vi "XP2i.vi"(4 "error in":T12, 7 "Command":T13) -> (0 "error out":T12, 3 "Response":T10)   [LabVIEW 2018]
uses:
  MOKO_LabViewLibrary/MokoLowLevel/MokoLowLovelControl/MLLC_Command.ctl
  MOKO_LabViewLibrary/MokoLowLevel/MokoLowLovelControl/MLLC_Error.ctl
  MOKO_LabViewLibrary/MokoLowLevel/MokoLowLovelControl/MLLC_Mode.ctl
  MOKO_LabViewLibrary/MokoLowLevel/MokoLowLovelControl/MLLC_Response.ctl
  MOKO_LabViewLibrary/MokoLowLevel/MokoLowLovelControl/MLLC_DriverName.ctl
  MOKO_LabViewLibrary/MokoLowLevel/MokoLowLovelControl/MLLC_ResponseInit.ctl
  MOKO_LabViewLibrary/MokoLowLevel/MokoLowLovelControl/MLLC_Request.ctl
  MOKO_LabViewLibrary/MokoLowLevel/MokoLowLovelControl/MLLC_ErrorCode.ctl
  MOKO_LabViewLibrary/MokoLowLevel/MokoLowLovelControl/MLLC_DriverConnectCluster.ctl
  MOKO_LabViewLibrary/MokoLowLevel/MokoLowLovelControl/MLLC_InterfaceType.ctl
  MOKO_LabViewLibrary/MokoLowLevel/MokoLowLovelControl/MLLC_OpenedSession.ctl
  MOKO_LabViewLibrary/MokoLowLevel/MokoLowLovelControl/MLLC_InterfaceSettings.ctl
  MOKO_LabViewLibrary/MokoLowLevel/MokoLowLovelControl/MLLC_InterfaceKind.ctl
  MOKO_LabViewLibrary/MokoLowLevel/MokoLowLovelControl/MLLC_Rs232Settings.ctl
panel:
  in  "DriverSettings":cluster{"DriverConnect":T1}={"DriverConnect"={"InterfaceType"=enum."VISA", "OpenedSession"="COM4", "InterfaceSettings"={"Interface"=enum."RS232", "EOS 4 read"=enum."Default (=EOS 4 write)", "EOS 4 write"=enum."CR (\\r)", "TMO, ms"=2000, "Sett"=variant(cluster{"Baud Rate":u32, "Data Bits":u16, "Parity":u16, "Stop Bits":u16, "Flow Control":u16, "Eho":bool} {"Baud Rate"=75, "Data Bits"=0, "Parity"=0, "Stop Bits"=0, "Flow Control"=0, "Eho"=FALSE})}}}
  in  "Error Code":T6=5420
  in  "Request":T7="?MOD"
  in  "ResponseInit":T8="XP2I"
  in  "Driver Name":T9="Crystal XP2"
  in  "Mode":T11=enum."Check"
  # "XP2i"
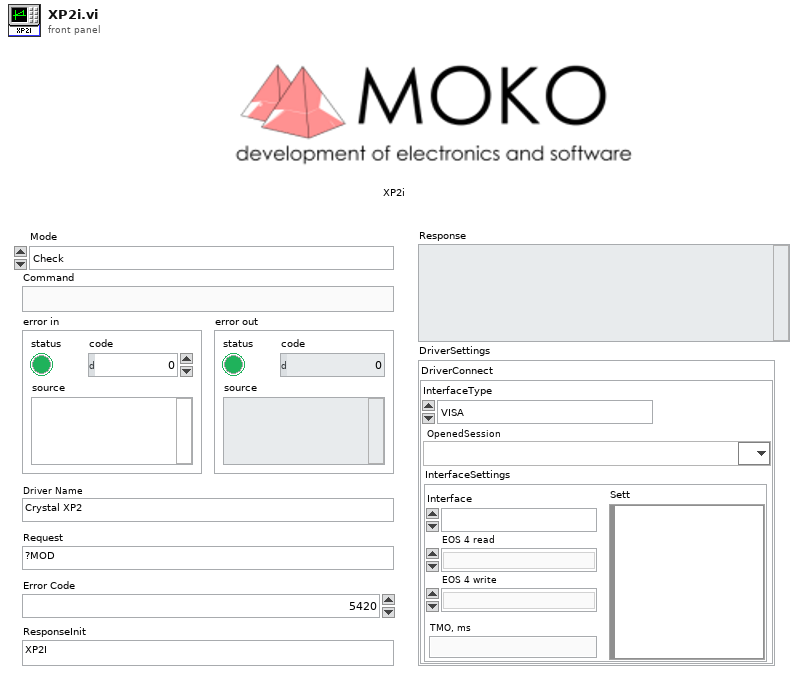
[diagram p1: front panel]
types:
  T1 = typedef "MLLC_DriverConnectCluster.ctl" = cluster{"InterfaceType":T2, "OpenedSession":T3, "InterfaceSettings":T4}
  T2 = typedef "MLLC_InterfaceType.ctl" = enum16{"VISA", "Prologix USB-GPIB"}
  T3 = typedef "MLLC_OpenedSession.ctl" = refnum<visa-resource-name>
  T4 = typedef "MLLC_InterfaceSettings.ctl" = cluster{"Interface":T5, "EOS 4 read":enum16{"Default (=EOS 4 write)", "CR (\\r)", "LF (\\n)", "None"}, "EOS 4 write":enum16{"CR+LF (\\r\\n)", "CR (\\r)", "LF (\\n)", "None"}, "TMO, ms":i32, "Sett":variant}
  T5 = typedef "MLLC_InterfaceKind.ctl" = enum16{"RS232", "GPIB", "USB", "Ethernet", "another"}
  T6 = typedef "MLLC_ErrorCode.ctl" = u32
  T7 = typedef "MLLC_Request.ctl" = string
  T8 = typedef "MLLC_ResponseInit.ctl" = string
  T9 = typedef "MLLC_DriverName.ctl" = string
  T10 = typedef "MLLC_Response.ctl" = string
  T11 = typedef "MLLC_Mode.ctl" = enum16{"get", "set", "close", "Init", "Check"}
  T12 = typedef "MLLC_Error.ctl" = errorcluster
  T13 = typedef "MLLC_Command.ctl" = string
  T14 = typedef "MLLC_Rs232Settings.ctl" = cluster{"Baud Rate":u32, "Data Bits":u16, "Parity":u16, "Stop Bits":u16, "Flow Control":u16, "Eho":bool}
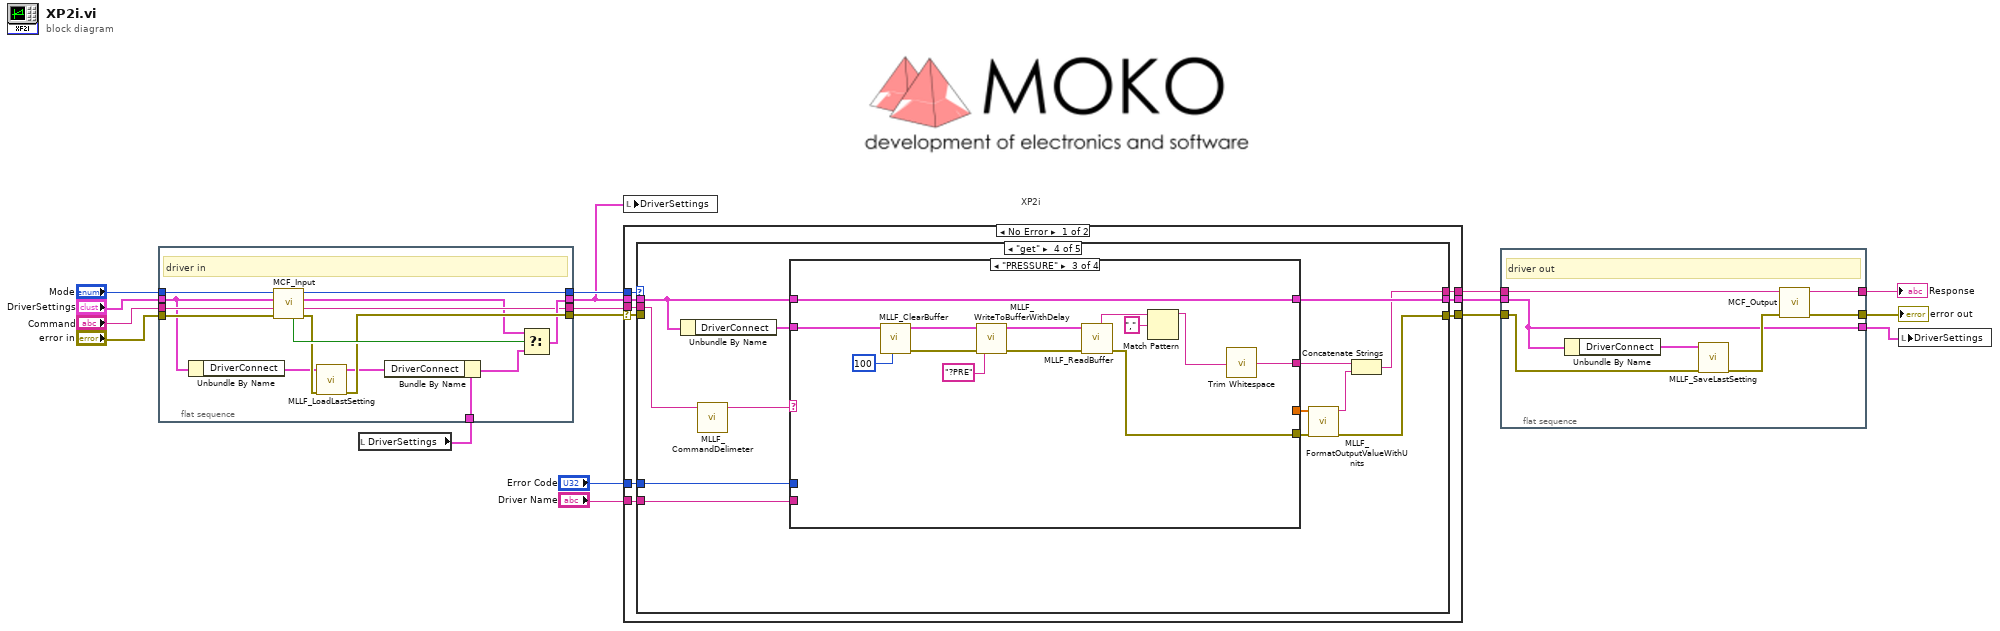
[diagram p0: block diagram]
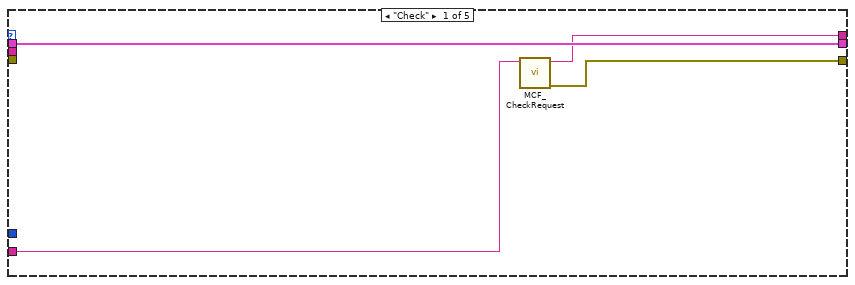
[diagram p2: hidden frame]
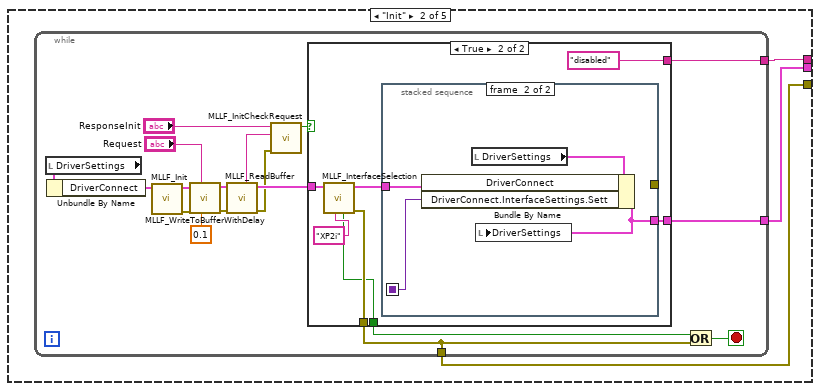
[diagram p3: hidden frame]
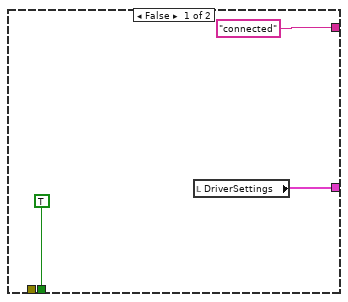
[diagram p4: hidden frame]
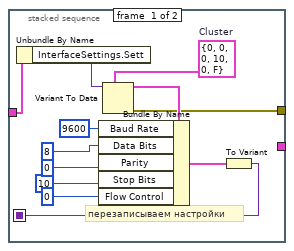
[diagram p5: hidden frame]
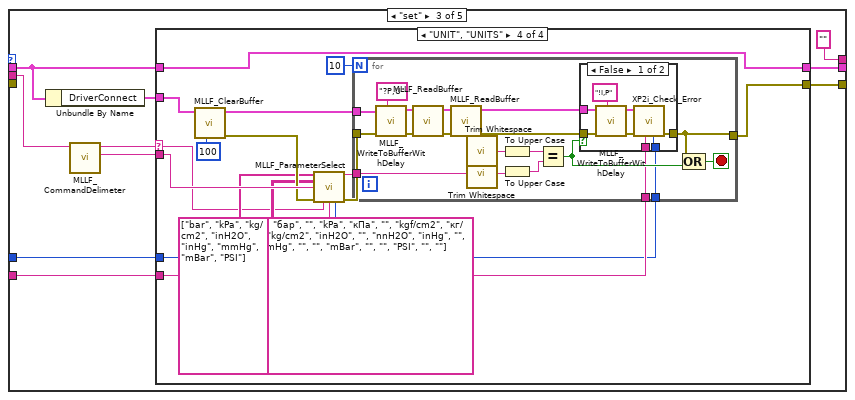
[diagram p6: hidden frame]
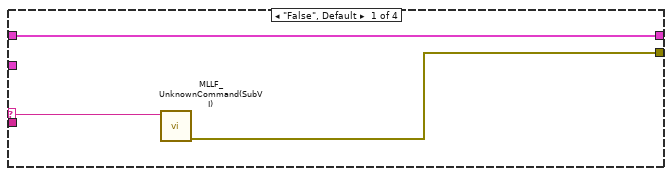
[diagram p7: hidden frame]
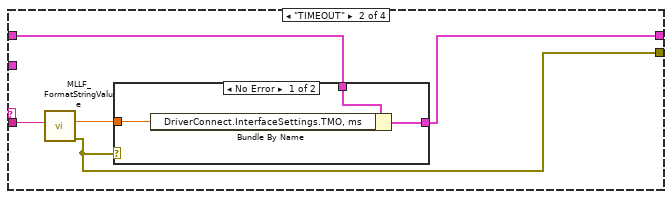
[diagram p8: hidden frame]
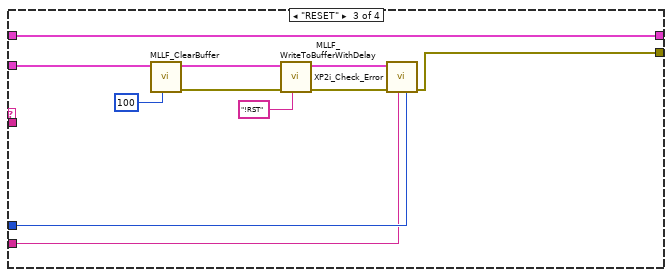
[diagram p10: hidden frame]
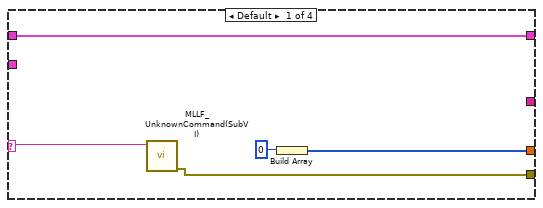
[diagram p12: hidden frame]
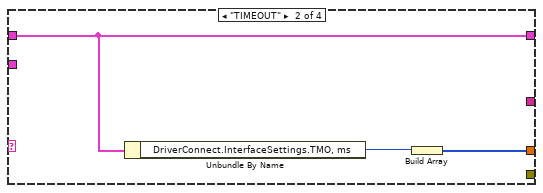
[diagram p13: hidden frame]
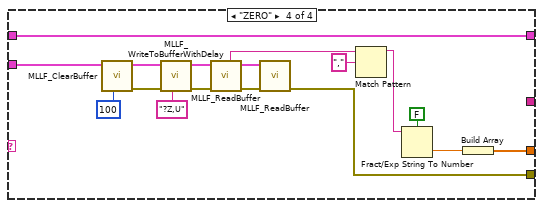
[diagram p14: hidden frame]
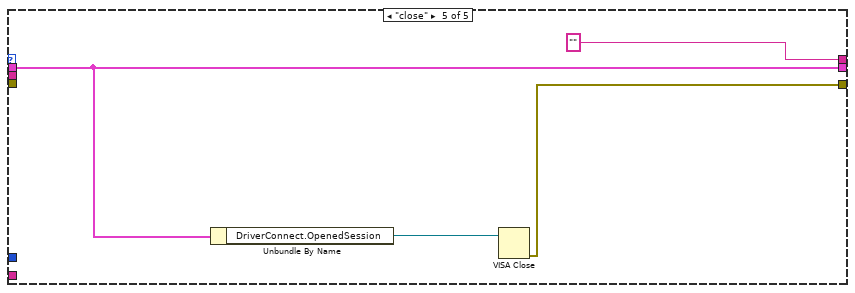
[diagram p15: hidden frame]
diagram:
  # "XP2i"
  n1 = flat-sequence {
    tunnel: [w26] -> w9
    tunnel: [w31] -> w11
    tunnel: "Command" -> [w28]
    tunnel: "Mode" -> [w30]
    tunnel: "DriverSettings" -> [w22]
    tunnel: w12 -> [w20]
    tunnel: "error in" -> [w25]
    tunnel: [w24] -> w10
    tunnel: [w23] -> w8
    frame #0 {
      # "driver in"
      n2 = Unbundle By Name(w22) -> ("DriverConnect"=w21:T1)
      n3 = call "MCF_Input.vi"("error in (no error)"=w25, "Command"=w28, "Mode"=w30) -> ("error out"=w27:errorcluster, "Command out"=w23:string, "Mode out"=w31:T11, "Boolean"=w29:bool)  [unwired: 5 in]
      n4 = call "MLLF_LoadLastSetting.vi"("Error In"=w27, "DriverConnectCluster in"=w21) -> ("Error Out"=w26:errorcluster, "DriverConnectCluster out"=w19:T1)  [unwired: 8 in]
      n5 = Bundle By Name(cluster=w20, "DriverConnect"=w19) -> (w18:cluster{"DriverConnect":T1})
      n6 = Select(t=w22, s=w29, f=w18) -> (s? t:f=w24:cluster{"DriverConnect":T1})
    }
  }
  n7 = local read "DriverSettings"() -> (w12:cluster{"DriverConnect":T1})
  n8 = local write "DriverSettings"(w10) -> ()
  n9 = case shown="No Error" w9 {
    selector: w9 -> [w37 w225]
    tunnel: [w32 w225] -> w1
    tunnel: w11 -> [w40 _]
    tunnel: [w39 _] -> w7
    tunnel: w8 -> [w38 _]
    tunnel: w10 -> [w34 w224]
    tunnel: "Error Code" -> [w36 _]
    tunnel: "Driver Name" -> [w35 _]
    tunnel: [w33 w224] -> w6
    frame No Error {
      n10 = case shown="\"get\"" w40 {
        tunnel: [w42 w47 "" ("Output String") w177 "" ("Output String")] -> w39
        tunnel: w38 -> [_ _ w94 w170 _]
        tunnel: w37 -> [_ _ _ _ _]
        tunnel: w36 -> [_ _ w101 w180 _]
        tunnel: w35 -> [w43 _ w98 w179 _]
        tunnel: w34 -> [w44 _ w100 w181 w222]
        tunnel: [w44 w46 w99 w178 w222] -> w33
        tunnel: [w41 w45 w97 w171 w221] -> w32
        frame "Check" {
          n11 = call "MCF_CheckRequest.vi"("Driver Name"=w43) -> ("Error Out"=w41:errorcluster, "Output String"=w42:string)  [unwired: 9 in]
        }
        frame "Init" {
          n12 = while {
            tunnel: [w60] -> w45
            tunnel: [w57] -> w47
            tunnel: [w56] -> w46
            stop <- w62 stop-if-true
            n13 = local read "DriverSettings"() -> (w50:cluster{"DriverConnect":T1})
            n14 = Unbundle By Name(w50) -> ("DriverConnect"=w49:T1)
            n15 = call "MLLF_Init.vi"("DriverConnect in"=w49) -> ("Error Out"=w64:errorcluster, "DriverConnect out"=w63:T1)  [unwired: 7 in]
            n16 = call "MLLF_WriteToBufferWithDelay.vi"("Delay Time ( 0,05 s)"=0.1 ("Delay Time (s)"), "Command"="Request", "Error In"=w64, "DriverConnect in"=w63) -> ("Error Out"=w59:errorcluster, "DriverConnect out"=w48:T1)  [unwired: 6 in]
            n17 = call "MLLF_ReadBuffer.vi"("Error In"=w59, "DriverConnect in"=w48) -> ("Error Out"=w54:errorcluster, "DriverConnect out"=w65:T1, "String"=w55:string)  [unwired: 6 in]
            n18 = call "MLLF_InitCheckRequest.vi"("error in (no error)"=w54, "Answer"=w55, "Response Init"="ResponseInit") -> ("Design"=w53:bool)  [unwired: 7 in, 1 out]
            n19 = case shown="True" w53 {
              tunnel: w65 -> [_ w74]
              tunnel: [TRUE w70] -> w61
              tunnel: [_ w75] -> w60
              tunnel: ["connected" "disabled"] -> w57
              tunnel: [w66 w69] -> w56
              frame False {
                n20 = local read "DriverSettings"() -> (w66:cluster{"DriverConnect":T1})
              }
              frame True {
                n21 = call "MLLF_InterfaceSelection.vi"("Driver Name"="XP2i" ("String"), "DriverConnect in"=w74) -> ("error out"=w75:T12, "DriverConnect out"=w73:T1, "stop init?"=w70:bool)  [unwired: 7 in]
                n22 = stacked-sequence {
                  seq-local: [w79 _] -> [_ w88]
                  tunnel: w73 -> [w77 w89]
                  tunnel: [w80 _] -> _
                  tunnel: [_ w90] -> w69
                  frame #0 {
                    w81 = T14 {"Baud Rate"=0, "Data Bits"=0, "Parity"=0, "Stop Bits"=10, "Flow Control"=0, "Eho"=FALSE}  # Cluster
                    # "перезаписываем настройки"
                    n23 = Unbundle By Name(w77) -> ("InterfaceSettings.Sett"=w76:variant)
                    n24 = Variant To Data(type=w81, Variant=w76) -> (data=w82:T14, error out=w80:errorcluster)  [unwired: 1 in]
                    n25 = Bundle By Name(cluster=w82, "Baud Rate"=u32 9600, "Data Bits"=u16 8 ("Serial Settings:Data Bits"), "Parity"=u16 0 ("Serial Settings:Parity"), "Stop Bits"=u16 10 ("Serial Settings:Stop Bits"), "Flow Control"=u16 0 ("Serial Settings:Flow Control")) -> (w87:T14)
                    n26 = To Variant(anything=w87) -> (Variant=w79:variant)
                  }
                  frame #1 {
                    n27 = local read "DriverSettings"() -> (w91:cluster{"DriverConnect":T1})
                    n28 = Bundle By Name(cluster=w91, "DriverConnect"=w89, "DriverConnect.InterfaceSettings.Sett"=w88) -> (w90:cluster{"DriverConnect":T1})
                    n29 = local write "DriverSettings"(w90) -> ()
                  }
                }
              }
            }
            n30 = Or(x=w61, y=w60) -> (x .or. y?=w62:bool)
          }
        }
        frame "set" {
          n31 = Unbundle By Name(w100) -> ("DriverConnect"=w95:T1)
          n32 = call "MLLF_CommandDelimeter.vi"("command with param"=w94) -> ("param 1"=w92:string, "command"=w93:string)  [unwired: 7 in, 2 out]
          n33 = case shown="\"UNIT\", \"UNITS\"" w93 {
            selector: w93 -> [w103 _ _ w125]
            tunnel: w92 -> [_ w107 _ w137]
            tunnel: w101 -> [_ _ w122 w135]
            tunnel: w100 -> [w104 w108 w124 w128]
            tunnel: [w104 w109 w124 w128] -> w99
            tunnel: w98 -> [_ _ w121 w136]
            tunnel: w95 -> [_ _ w115 w127]
            tunnel: [w102 w105 w114 w126] -> w97
            frame "False", Default {
              n34 = call "MLLF_UnknownCommand(SubVI).vi"("Unknown command"=w103) -> ("error out"=w102:errorcluster)  [unwired: 10 in]
            }
            frame "TIMEOUT" {
              n35 = call "MLLF_FormatStringValue.vi"("String Value"=w107) -> ("error out"=w105:T12, "number"=w106:dbl)  [unwired: 8 in, 1 out]
              n36 = case shown="No Error" w105 {
                tunnel: [w112 w113] -> w109
                tunnel: w108 -> [w111 w113]
                tunnel: w106 -> [w110 _]
                frame No Error {
                  n37 = Bundle By Name(cluster=w111, "DriverConnect.InterfaceSettings.TMO, ms"=w110) -> (w112:cluster{"DriverConnect":T1})
                }
                frame Error {
                }
              }
            }
            frame "RESET" {
              n38 = call "MLLF_ClearBuffer.vi"("Timeout"=u32 100, "DriverConnect in"=w115) -> ("Error Out"=w119:errorcluster, "DriverConnect out"=w118:T1)  [unwired: 6 in, 1 out]
              n39 = call "MLLF_WriteToBufferWithDelay.vi"("Command"="!RST" ("String"), "Error In"=w119, "DriverConnect in"=w118) -> ("Error Out"=w117:errorcluster, "DriverConnect out"=w123:T1)  [unwired: 7 in]
              n40 = call "XP2i_Check_Error.vi"("Error Code"=w122, "Driver Name"=w121, "Error In"=w117, "DriverConnect in"=w123) -> ("Error Out"=w114:errorcluster)  [unwired: 6 in, 1 out]
            }
            frame "UNIT", "UNITS" {
              n41 = call "MLLF_ClearBuffer.vi"("Timeout"=u32 100, "DriverConnect in"=w127) -> ("Error Out"=w134:errorcluster, "DriverConnect out"=w138:T1)  [unwired: 6 in, 1 out]
              n42 = call "MLLF_ParameterSelect.vi"("Command to equipment"=string[] ["bar", "kPa", "kg/cm2", "inH2O", "inHg", "mmHg", "mBar", "PSI"] ("Parameters 2 equipment"), "Names"=string[][] [["bar", "бар", ""], ["kPa", "кПа", ""], ["kgf/cm2", "кг/см2", "kg/cm2"], ["inH2O", "", "nnH2O"], ["inHg", "", ""], ["mmHg", "", ""], ["mBar", "", ""], ["PSI", "", ""]], "Input"=w137, "Error In"=w134, "Command"=w125, "Driver Name"=w136, "Error Code"=w135) -> ("Choice"=w132:string, "Error Out"=w133:errorcluster)  [unwired: 7 in]
              n43 = for {
                N: 10 -> [_]
                tunnel: w138 -> [w149]
                tunnel: [w143] -> w126
                tunnel: w132 -> [w147]
                tunnel: w136 -> [w141]
                tunnel: w135 -> [w140]
                tunnel: w133 -> [w148]
                stop <- w155 stop-if-true
                n44 = call "MLLF_WriteToBufferWithDelay.vi"("Command"="?P,U" ("String"), "Error In"=w148, "DriverConnect in"=w149) -> ("Error Out"=w151:errorcluster, "DriverConnect out"=w158:T1)  [unwired: 7 in]
                n45 = call "MLLF_ReadBuffer.vi"("Error In"=w151, "DriverConnect in"=w158) -> ("Error Out"=w154:errorcluster, "DriverConnect out"=w153:T1)  [unwired: 6 in, 1 out]
                n46 = call "MLLF_ReadBuffer.vi"("Error In"=w154, "DriverConnect in"=w153) -> ("Error Out"=w144:errorcluster, "DriverConnect out"=w145:T1, "String"=w152:string)  [unwired: 6 in]
                n47 = call <vilib>:"Trim Whitespace.vi"("string"=w152) -> ("trimmed string"=w150:string)  [unwired: 1 in]
                n48 = call <vilib>:"Trim Whitespace.vi"("string"=w147) -> ("trimmed string"=w146:string)  [unwired: 1 in]
                n49 = To Upper Case(1:w150) -> (0:w157:string)
                n50 = To Upper Case(1:w146) -> (0:w156:string)
                n51 = Equal?(x=w157, y=w156) -> (x = y?=w142:bool)
                n52 = case shown="False" w142 {
                  tunnel: w145 -> [w164 _]
                  tunnel: w144 -> [w163 w168]
                  tunnel: [w162 w168] -> w143
                  tunnel: w141 -> [w161 _]
                  tunnel: w140 -> [w160 _]
                  frame False {
                    n53 = call "MLLF_WriteToBufferWithDelay.vi"("Command"="!I,P" ("String"), "Error In"=w163, "DriverConnect in"=w164) -> ("Error Out"=w165:errorcluster, "DriverConnect out"=w166:T1)  [unwired: 7 in]
                    n54 = call "XP2i_Check_Error.vi"("Error Code"=w160, "Driver Name"=w161, "Error In"=w165, "DriverConnect in"=w166) -> ("Error Out"=w162:errorcluster)  [unwired: 6 in, 1 out]
                  }
                  frame True {
                  }
                }
                n55 = Compound Arithmetic op=OR(w143, w142) -> (w155:bool)
              }
            }
          }
        }
        frame "get" {
          n56 = Unbundle By Name(w181) -> ("DriverConnect"=w172:T1)
          n57 = call "MLLF_CommandDelimeter.vi"("command with param"=w170) -> ("command"=w169:string)  [unwired: 7 in, 3 out]
          n58 = case shown="\"PRESSURE\"" w169 {
            selector: w169 -> [w183 _ _ _]
            tunnel: [w182 _ w198 w212] -> w176
            tunnel: w180 -> [_ _ _ _]
            tunnel: [w186 w189 w202 w219] -> w178
            tunnel: w181 -> [w186 w189 w202 w219]
            tunnel: [w184 w187 _ w216] -> w175
            tunnel: w179 -> [_ _ _ _]
            tunnel: [_ _ w193 _] -> w173
            tunnel: w172 -> [_ _ w190 w203]
            frame Default {
              n59 = call "MLLF_UnknownCommand(SubVI).vi"("Unknown command"=w183) -> ("error out"=w182:errorcluster)  [unwired: 10 in]
              n60 = Build Array(0 ("TimeOut")) -> (w184:i32[])
            }
            frame "TIMEOUT" {
              n61 = Unbundle By Name(w189) -> ("DriverConnect.InterfaceSettings.TMO, ms"=w188:i32)
              n62 = Build Array(w188) -> (w187:i32[])
            }
            frame "PRESSURE" {
              n63 = call "MLLF_ClearBuffer.vi"("Timeout"=u32 100, "DriverConnect in"=w190) -> ("Error Out"=w199:errorcluster, "DriverConnect out"=w200:T1)  [unwired: 6 in, 1 out]
              n64 = call "MLLF_WriteToBufferWithDelay.vi"("Command"="?PRE" ("String"), "Error In"=w199, "DriverConnect in"=w200) -> ("Error Out"=w192:errorcluster, "DriverConnect out"=w197:T1)  [unwired: 7 in]
              n65 = call "MLLF_ReadBuffer.vi"("Error In"=w192, "DriverConnect in"=w197) -> ("Error Out"=w198:errorcluster, "String"=w196:string)  [unwired: 6 in, 1 out]
              n66 = Match Pattern(string=w196, regular expression=",") -> (before substring=w194:string)  [unwired: 1 in, 3 out]
              n67 = call <vilib>:"Trim Whitespace.vi"("string"=w194) -> ("trimmed string"=w193:string)  [unwired: 1 in]
            }
            frame "ZERO" {
              n68 = call "MLLF_ClearBuffer.vi"("Timeout"=u32 100, "DriverConnect in"=w203) -> ("Error Out"=w213:errorcluster, "DriverConnect out"=w214:T1)  [unwired: 6 in, 1 out]
              n69 = call "MLLF_WriteToBufferWithDelay.vi"("Command"="?Z,U" ("String"), "Error In"=w213, "DriverConnect in"=w214) -> ("Error Out"=w205:errorcluster, "DriverConnect out"=w209:T1)  [unwired: 7 in]
              n70 = call "MLLF_ReadBuffer.vi"("Error In"=w205, "DriverConnect in"=w209) -> ("Error Out"=w208:errorcluster, "DriverConnect out"=w207:T1, "String"=w206:string)  [unwired: 6 in]
              n71 = call "MLLF_ReadBuffer.vi"("Error In"=w208, "DriverConnect in"=w207) -> ("Error Out"=w212:errorcluster)  [unwired: 6 in, 2 out]
              n72 = Match Pattern(string=w206, regular expression=",") -> (before substring=w210:string)  [unwired: 1 in, 3 out]
              n73 = Fract/Exp String To Number(use system decimal point (T)=FALSE, string=w210) -> (number=w217:dbl)  [unwired: 2 in, 1 out]
              n74 = Build Array(w217) -> (w216:dbl[])
            }
          }
          n75 = call "MLLF_FormatOutputValueWithUnits.vi"("error in"=w176, "ValuesIn"=w175) -> ("error out"=w171:T12, "Result string"=w174:T13)  [unwired: 8 in]
          n76 = Concatenate Strings(w173, w174) -> (w177:string)
        }
        frame "close" {
          n77 = Unbundle By Name(w222) -> ("DriverConnect.OpenedSession"=w223:T3)
          n78 = VISA Close(VISA resource name=w223) -> (error out=w221:errorcluster)  [unwired: 1 in]
        }
      }
    }
    frame Error {
    }
  }
  n79 = flat-sequence {
    tunnel: [w232] -> w5
    tunnel: w7 -> [w231]
    tunnel: w1 -> [w228]
    tunnel: w6 -> [w227]
    tunnel: [w227] -> w4
    tunnel: [w229] -> w3
    frame #0 {
      # "driver out"
      n80 = Unbundle By Name(w227) -> ("DriverConnect"=w226:T1)
      n81 = call "MLLF_SaveLastSetting.vi"("error in"=w228, "DriverConnectCluster in"=w226) -> ("error out"=w230:T12)  [unwired: 8 in, 1 out]
      n82 = call "MCF_Output.vi"("Error In"=w230, "Input"=w231) -> ("Error Out"=w229:errorcluster, "Output"=w232:string)  [unwired: 8 in]
    }
  }
  n83 = local write "DriverSettings"(w4) -> ()
  "error out" <- w3
  "Response" <- w5
